vi "Enqueue Logs Element.vi"(8 "Error In":errorcluster, 9 "Timeout":i32, 10 "Event Occured":refnum<class "EventsAbstract.lvclass">, 11 "EventLog in":refnum<class "ErrorLog.lvclass">) -> (0 "Error Out":errorcluster, 1 "Timed out?":bool, 3 "EventLog out":refnum<class "ErrorLog.lvclass">)   [LabVIEW 2019, in "ErrorLog.lvlib" / "ErrorLog.lvclass"]
uses:
  ErrorLog.lvclass
  Classes/EventsAbstract/EventsAbstract.lvclass
  Classes/Error/Error.lvclass
  ErrorLog.lvclass/ErrorLog.ctl
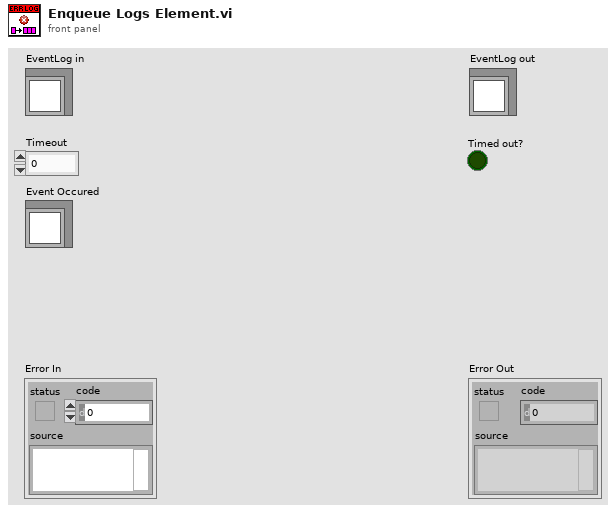
[diagram p1: front panel]
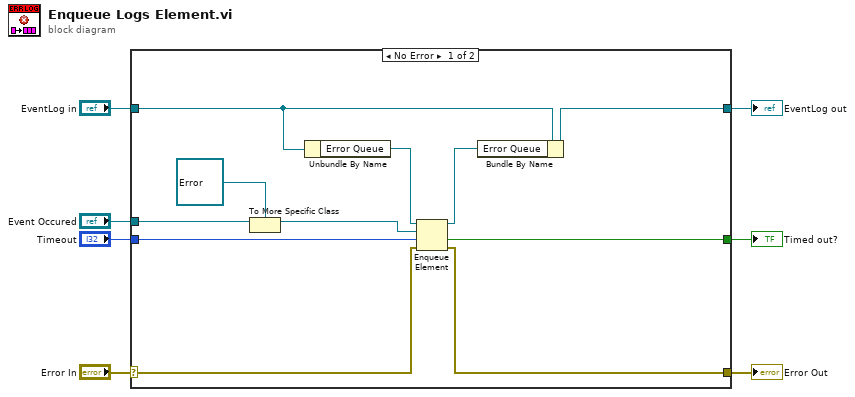
[diagram p0: block diagram]
diagram:
  n1 = case shown="No Error" "Error In" {
    selector: "Error In" -> [w17 w20]
    tunnel: [w13 w20] -> w7
    tunnel: [w16 w19] -> w5
    tunnel: "EventLog in" -> [w18 w19]
    tunnel: [w14 _] -> w6
    tunnel: "Timeout" -> [w15 _]
    tunnel: "Event Occured" -> [w12 _]
    frame No Error {
      n2 = To More Specific Class(target class=refnum<class "Error.lvclass"> refnum ("Error.lvclass"), reference=w12) -> (specific class reference=w9:refnum<class "Error.lvclass">)  [unwired: 1 in, 1 out]
      n3 = Unbundle By Name(w18) -> ("Error Queue"=w11:refnum<queue>)
      n4 = Enqueue Element(queue=w11, element=w9, timeout in ms (-1)=w15, error in (no error)=w17) -> (queue out=w10:refnum<queue>, timed out?=w14:bool, error out=w13:errorcluster)
      n5 = Bundle By Name(cluster=w18, "Error Queue"=w10) -> (w16:refnum<class "ErrorLog.lvclass">)
    }
    frame Error {
    }
  }
  "Error Out" <- w7
  "EventLog out" <- w5
  "Timed out?" <- w6
